vi "User Function.vi"(6 "expression (\"VI\") (max 58 chars)":string="VI", 7 "unit (optional)":string, 8 "error in (no error)":errorcluster, 9 "function name (\"UFUN1\") (max 6 chars)":string="UFUN1", 10 "operation":i32(slide) max=3 scale=0.0..3.0, 11 "VISA session":refnum<visa-resource-name>) -> (0 "error out":errorcluster, 1 "currently defined user functions":string, 3 "VISA resource name out":refnum<visa-resource-name>)   [LabVIEW 2016, in "Agilent 415X Series.lvlib"]
doc: "In this VI, you define/delete/list user functions. For details about user functions, refer to \"User Function\" in Chapter 6 of User's Dictionary Reference.\n\n* This VI does NOT perform any error checking on the control settings. That is, this VI does not check the length of UNIT or NAME, nor does it verify the existence of variables used in EXPRESSION. Entering a string longer than allowed will cause an error to be placed in the instrument's error queue. To read the error queue, run HP415xA Sys-Report Error.vi. An invalid expression will return an error when you switch from user function definition to other pages (sub-systems)."
uses:
  Agilent 415X Series.lvlib
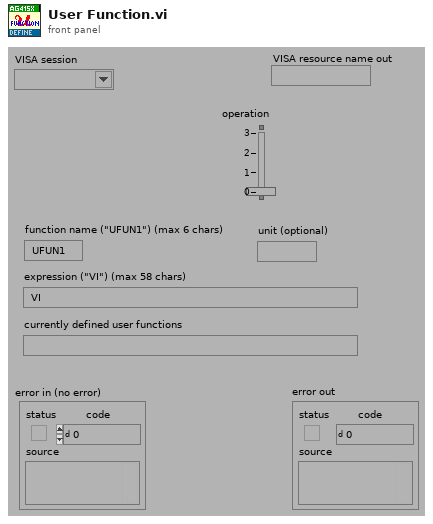
[diagram p1: front panel]
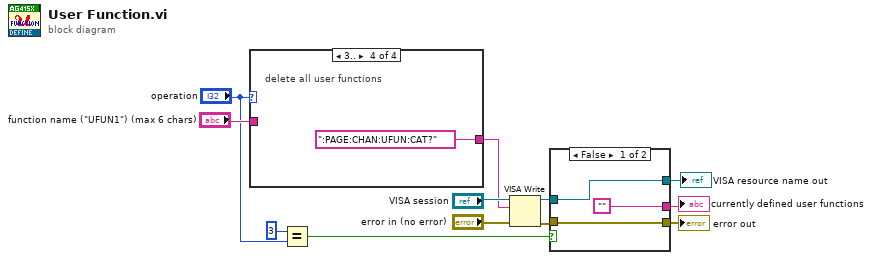
[diagram p0: block diagram]
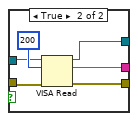
[diagram p2: hidden frame]
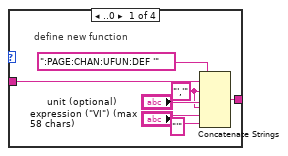
[diagram p3: hidden frame]
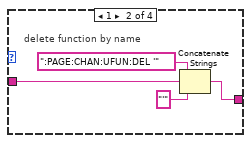
[diagram p4: hidden frame]
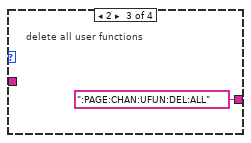
[diagram p5: hidden frame]
diagram:
  n1 = case shown="3.." "operation" {
    tunnel: [w14 w22 ":PAGE:CHAN:UFUN:DEL:ALL" ":PAGE:CHAN:UFUN:CAT?"] -> w9
    tunnel: "function name (\"UFUN1\") (max 6 chars)" -> [w13 w20 _ _]
    frame ..0 {
      w17 = "','"
      # "define new function"
      n2 = Concatenate Strings(":PAGE:CHAN:UFUN:DEF '", w13, w17, "unit (optional)", w17, "expression (\"VI\") (max 58 chars)", "'") -> (w14:string)
    }
    frame 1 {
      # "delete function by name"
      n3 = Concatenate Strings(":PAGE:CHAN:UFUN:DEL '", w20, "'") -> (w22:string)
    }
    frame 2 {
      # "delete all user functions"
    }
    frame 3.. {
      # "delete all user functions"
    }
  }
  n4 = Equal?(x=3, y="operation") -> (x = y?=w3:bool)
  n5 = VISA Write(VISA resource name="VISA session", write buffer=w9, error in (no error)="error in (no error)") -> (VISA resource name out=w8:refnum<visa-resource-name>, error out=w7:errorcluster)  [unwired: 1 out]
  n6 = case shown="False" w3 {
    tunnel: w8 -> [w26 w33]
    tunnel: w7 -> [w27 w32]
    tunnel: [w27 w31] -> w6
    tunnel: ["" ("Empty String Constant") w30] -> w5
    tunnel: [w26 w29] -> w1
    frame False {
    }
    frame True {
      n7 = VISA Read(VISA resource name=w33, byte count=u32 200, error in (no error)=w32) -> (VISA resource name out=w29:refnum<visa-resource-name>, read buffer=w30:string, error out=w31:errorcluster)  [unwired: 1 out]
    }
  }
  "error out" <- w6
  "currently defined user functions" <- w5
  "VISA resource name out" <- w1
